vi "Status Message_Record.vi"(7 "QRD":T1, 8 "error in":errorcluster, 11 "Status Message":string) -> (0 "error out":errorcluster, 3 "Status Message Out":string, 5 "QRD Out":T1)   [LabVIEW 2025]
uses:
  Controls/Queues-Refs-Data.ctl
  Builds/Queue Wrappers.lvlibp/Q Packet.ctl
  Builds/Queue Wrappers.lvlibp
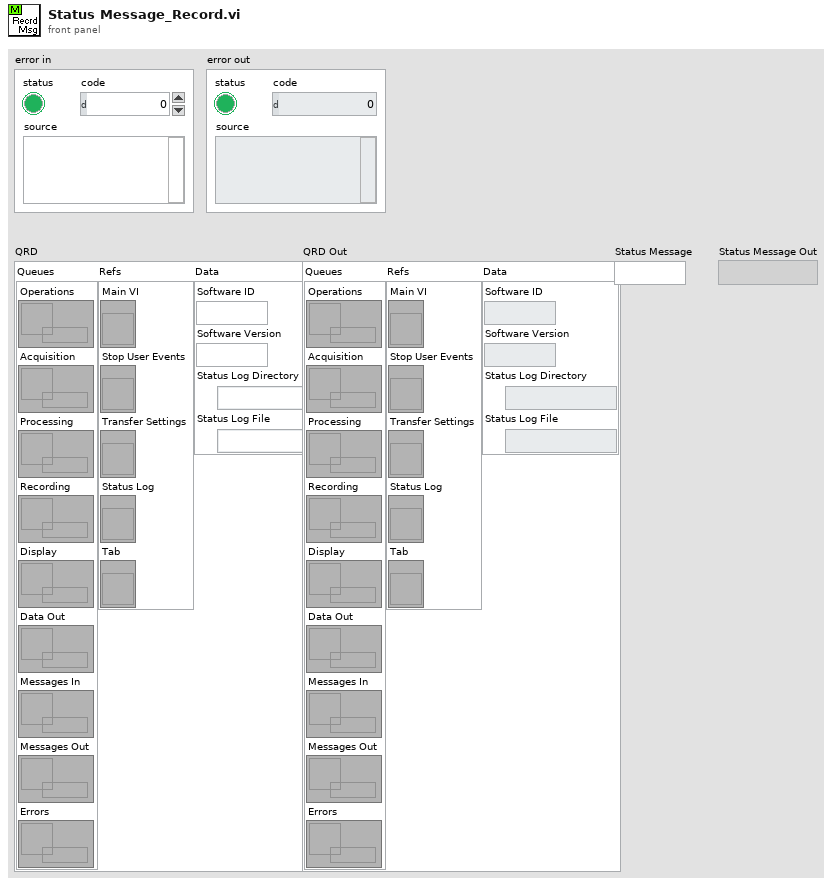
[diagram p1: front panel]
types:
  T1 = typedef "Queues-Refs-Data.ctl" = cluster{"Queues":cluster{"Operations":refnum<queue>, "Acquisition":refnum<queue>, "Processing":refnum<queue>, "Recording":refnum<queue>, "Display":refnum<queue>, "Data Out":refnum<queue>, "Messages In":refnum<queue>, "Messages Out":refnum<queue>, "Errors":refnum<queue>}, "Refs":cluster{"Main VI":refnum<vi>, "Stop User Events":refnum<vi>, "Transfer Settings":refnum<vi>, "Status Log":refnum<vi>, "Tab":refnum<vi>}, "Data":cluster{"Software ID":string, "Software Version":string, "Status Log Directory":path, "Status Log File":path}}
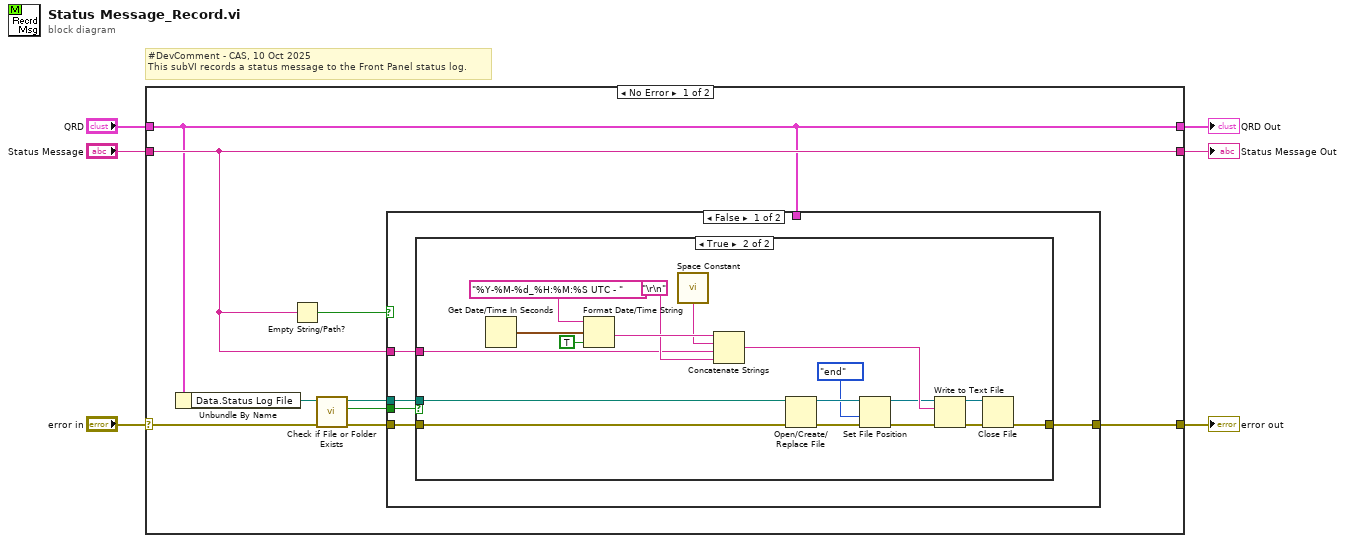
[diagram p0: block diagram]
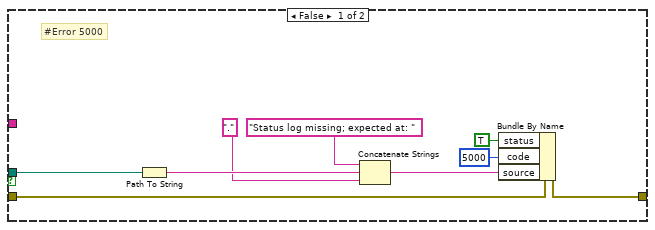
[diagram p2: hidden frame]
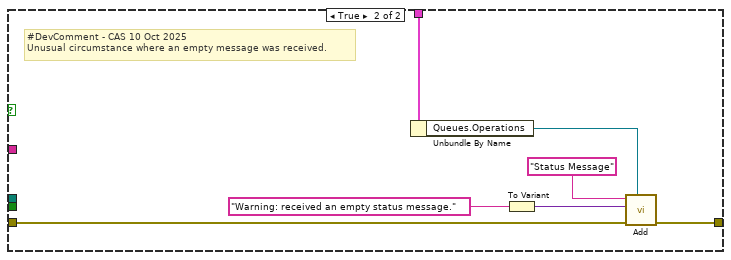
[diagram p3: hidden frame]
diagram:
  # "#DevComment - CAS, 10 Oct 2025\nThis subVI records a status message to the Front Panel status log."
  n1 = case shown="No Error" "error in" {
    selector: "error in" -> [w15 w56]
    tunnel: "QRD" -> [w7 w57]
    tunnel: [w7 w57] -> w5
    tunnel: [w11 w56] -> w4
    tunnel: "Status Message" -> [w8 w55]
    tunnel: [w8 w55] -> w1
    frame No Error {
      n2 = Unbundle By Name(w7) -> ("Data.Status Log File"=w14:path)
      n3 = Empty String/Path?(string/path=w8) -> (empty?=w10:bool)
      n4 = call <vilib>:"Check if File or Folder Exists.vi"("error in (no error)"=w15, "path"=w14) -> ("error out"=w12:errorcluster, "file or folder exists?"=w9:bool, "dup path"=w13:path)  [unwired: 7 in]
      n5 = case shown="False" w10 {
        tunnel: w13 -> [w20 _]
        tunnel: w12 -> [w19 w54]
        tunnel: [w18 w53] -> w11
        tunnel: w9 -> [w17 _]
        tunnel: w8 -> [w16 _]
        tunnel: w7 -> [_ w52]
        frame False {
          n6 = case shown="True" w17 {
            tunnel: w20 -> [w21 w38]
            tunnel: w19 -> [w23 w40]
            tunnel: [w22 w39] -> w18
            tunnel: w16 -> [_ w34]
            frame False {
              # "#Error 5000"
              n7 = Path To String(path=w21) -> (string=w28:string)
              n8 = Concatenate Strings("Status log missing; expected at: " ("source"), w28, "." ("string")) -> (w29:string)
              n9 = Bundle By Name(cluster=w23, "status"=TRUE, "code"=5000, "source"=w29) -> (w22:errorcluster)
            }
            frame True {
              n10 = Get Date/Time In Seconds() -> (seconds since 1Jan1904=w47:timestamp)
              n11 = Format Date/Time String(time format string (%c)="%Y-%M-%d_%H:%M:%S UTC - ", seconds (now)=w47, UTC format=TRUE) -> (date/time string=w44:string)
              n12 = call <vilib>:"Space Constant.vi"() -> ("String"=w43:string)
              n13 = Concatenate Strings(w44, w43, w34, "\r\n") -> (w37:string)
              n14 = Open/Create/Replace File(file path (use dialog)=w38, error in=w40) -> (refnum out=w36:refnum<file>, error out=w31:errorcluster)  [unwired: 4 in, 1 out]
              n15 = Set File Position(refnum=w36, from (0:start)=enum16{"start", "end", "current"}."end", error in=w31) -> (refnum out=w33:refnum<file>, error out=w30:errorcluster)  [unwired: 1 in]
              n16 = Write to Text File(file (use dialog)=w33, text=w37, error in=w30) -> (refnum out=w35:refnum<file>, error out=w41:errorcluster)  [unwired: 1 in, 1 out]
              n17 = Close File(refnum=w35, error in=w41) -> (error out=w39:errorcluster)  [unwired: 1 out]
            }
          }
        }
        frame True {
          # "#DevComment - CAS 10 Oct 2025\nUnusual circumstance where an empty message was received."
          n18 = Unbundle By Name(w52) -> ("Queues.Operations"=w51:refnum<queue>)
          n19 = To Variant(anything="Warning: received an empty status message." ("Packet ID")) -> (Variant=w48:variant)
          n20 = call "Add.vi"("Q Ref In"=w51, "error in"=w54, "Payload"=w48, "Packet ID"="Status Message") -> ("error out"=w53:errorcluster)  [unwired: 4 in, 3 out]
        }
      }
    }
    frame Error {
    }
  }
  "error out" <- w4
  "QRD Out" <- w5
  "Status Message Out" <- w1
